vi "19.6-DirectIIR-2nd Order.vi"() -> ()   [LabVIEW 2020]
doc: "Uses the Median Filter VI to analyze pulses in the presence of noise. The example generates a pulse contaminated with Gaussian noise and applies a median filter. For comparison purposes, the VI computes the pulse parameters of the filtered pulse."
uses:
  <vilib>/Analysis/3filter.llb/IIR Filter (DBL).vi
  <vilib>/Analysis/NI_AALBase.lvlib
panel:
  out "Filtered2":dbl[](graph)
  out "H[k]2":dbl[](graph)
  in  "BW":dbl(slide)=6.090909090909091 scale=1.0..50.0
  in  "stop":bool
  out "Sig":dbl[](graph)
  in  "Fo":dbl(slide)=159.58441558441558 scale=0.0..512.0
  out "Filtered1":dbl[](graph)
  out "H[k]1":dbl[](graph)
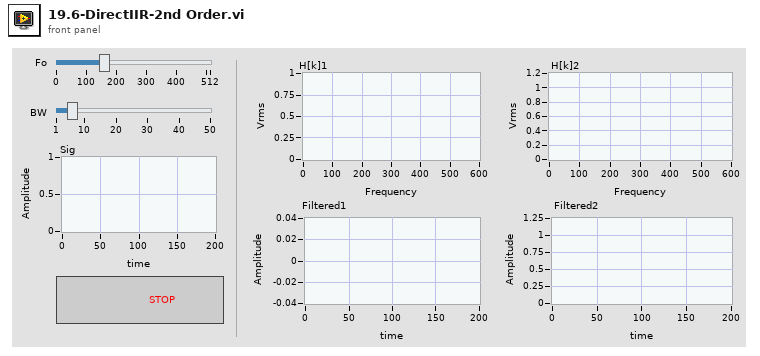
[diagram p1: front panel]
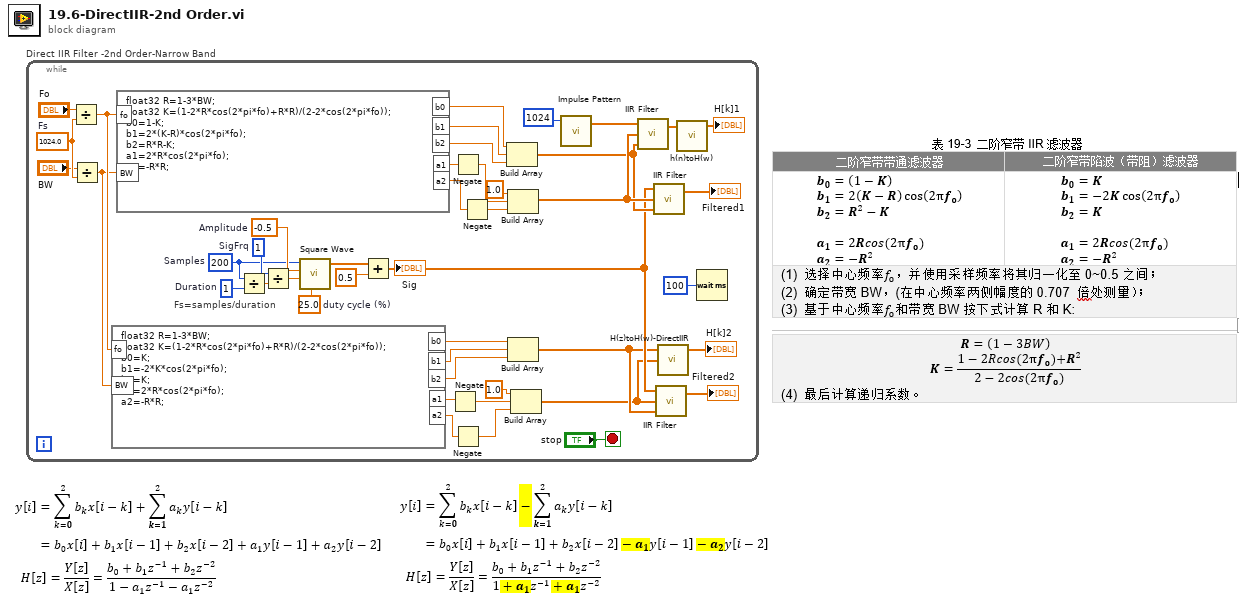
[diagram p0: block diagram]
diagram:
  n1 = while "Direct IIR Filter -2nd Order-Narrow Band" {
    stop <- "stop" stop-if-true
    w5 = 1024.0  # Fs
    w31 = 1  # Duration
    w42 = 1  # SigFrq
    w43 = 25.0  # duty cycle (%)
    w44 = -0.5  # Amplitude
    w33 = 200  # Samples
    # "Fs=samples/duration"
    n2 = Divide(x="Fo", y=w5) -> (x/y=w3:dbl)
    n3 = Divide(x="BW", y=w5) -> (x/y=w2:dbl)
    n4 = formula code="float32 R=1-3*BW;\nfloat32 K=(1-2*R*cos(2*pi*fo)+R*R)/(2-2*cos(2*pi*fo));\nb0=K;\nb1=-2*K*cos(2*pi*fo);\nb2=K;\na1=2*R*cos(2*pi*fo);\na2=-R*R;"("fo"=w3, "BW"=w2) -> ("b0"=w16:dbl, "b1"=w15:dbl, "b2"=w14:dbl, "a1"=w18:dbl, "a2"=w17:dbl)
    n5 = formula code="float32 R=1-3*BW;\nfloat32 K=(1-2*R*cos(2*pi*fo)+R*R)/(2-2*cos(2*pi*fo));\nb0=1-K;\nb1=2*(K-R)*cos(2*pi*fo);\nb2=R*R-K;\na1=2*R*cos(2*pi*fo);\na2=-R*R;"("fo"=w3, "BW"=w2) -> ("b0"=w28:dbl, "b1"=w27:dbl, "b2"=w26:dbl, "a1"=w23:dbl, "a2"=w24:dbl)
    n6 = Divide(x=w33, y=w31) -> (x/y=w32:dbl)
    n7 = Divide(x=w42, y=w32) -> (x/y=w39:dbl)
    n8 = call <vilib>:"Square Wave.vi"("samples"=w33, "amplitude"=w44, "frequency"=w39, "duty cycle (%)"=w43) -> ("square wave"=w41:dbl[])  [unwired: 2 in, 2 out]
    n9 = Add(x=w41, y=0.5) -> (x+y=w13:dbl[])
    "Sig" <- w13
    n10 = Negate(x=w18) -> (-x=w8:dbl)
    n11 = Negate(x=w23) -> (-x=w22:dbl)
    n12 = Negate(x=w17) -> (-x=w7:dbl)
    n13 = Negate(x=w24) -> (-x=w25:dbl)
    n14 = Build Array(w28, w27, w26) -> (w19:dbl[])
    n15 = Build Array(1.0 ("element"), w22, w25) -> (w37:dbl[])
    n16 = Build Array(w16, w15, w14) -> (w12:dbl[])
    n17 = Build Array(1.0 ("element"), w8, w7) -> (w1:dbl[])
    n18 = call <vilib>:"Impulse Pattern.vi"("samples"=1024 ("FFT size")) -> ("Impulse Pattern"=w38:dbl[])  [unwired: 2 in, 1 out]
    n19 = call-poly <vilib>:"IIR Filter.vi"("Forward Coefficients"=w19, "Reverse Coefficients"=w37, "X"=w38) -> ("Filtered X"=w35:dbl[])  [unwired: 1 in, 1 out]
    n20 = call-poly <vilib>:"IIR Filter.vi"("Forward Coefficients"=w19, "Reverse Coefficients"=w37, "X"=w13) -> ("Filtered X"=→"Filtered1":dbl[])  [unwired: 1 in, 1 out]
    n21 = call-poly <vilib>:"IIR Filter.vi"("Forward Coefficients"=w12, "Reverse Coefficients"=w1, "X"=w13) -> ("Filtered X"=→"Filtered2":dbl[])  [unwired: 1 in, 1 out]
    n22 = call "H(z)toH(w)-DirectIIR.vi"("Reverse"=w1, "Forward"=w12) -> ("Mag H(w)"=→"H[k]2":dbl[])  [unwired: 1 in, 2 out]
    n23 = call "h(n)toH(w).vi"("h(n)"=w35) -> ("Mag H(w)"=→"H[k]1":dbl[])  [unwired: 1 in, 2 out]
    n24 = Wait (ms)(milliseconds to wait=u32 100) -> ()  [unwired: 1 out]
  }
